vi "Write filter.vi"(8 "error in (no error)":errorcluster, 10 "Switch.lvclass":refnum<class "Switch.lvclass">, 11 "CRDS in":refnum<class "CRDS.lvclass">) -> (0 "error out":errorcluster, 3 "CRDS out":refnum<class "CRDS.lvclass">)   [LabVIEW 2013, in "CRDS.lvclass"]
uses:
  CRDS.lvclass
  Switch/Switch.lvclass
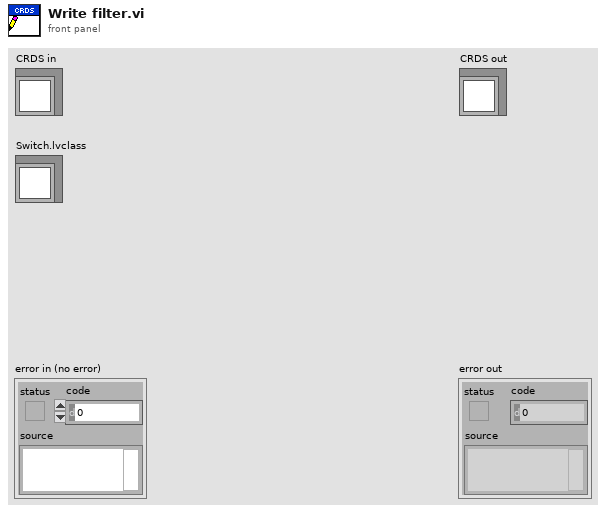
[diagram p1: front panel]
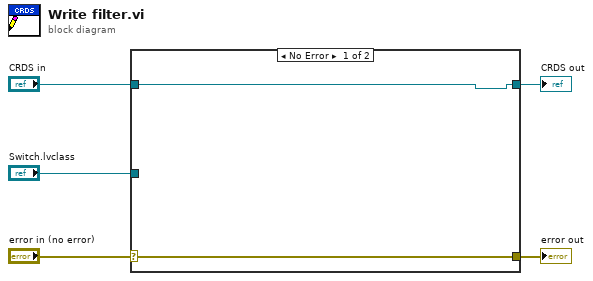
[diagram p0: block diagram]
diagram:
  n1 = case shown="No Error" "error in (no error)" {
    selector: "error in (no error)" -> [w7 w8]
    tunnel: [w7 w8] -> w4
    tunnel: [w6 w9] -> w2
    tunnel: "CRDS in" -> [w6 w9]
    tunnel: "Switch.lvclass" -> [_ _]
    frame No Error {
    }
    frame Error {
    }
  }
  "error out" <- w4
  "CRDS out" <- w2
